vi "Write CurrentLeftMostItem.vi"(8 "error in (no error)":errorcluster, 10 "CurrentLeftMostItem":i32, 11 "BreadcrumbNavigation in":refnum<class "BreadcrumbNavigator.lvclass">) -> (0 "error out":errorcluster, 3 "BreadcrumbNavigation out":refnum<class "BreadcrumbNavigator.lvclass">)   [LabVIEW 2015, in "BreadcrumbNavigator.lvclass"]
uses:
  BreadcrumbNavigator.lvclass
  BreadcrumbNavigator.lvclass/BreadcrumbNavigator.ctl
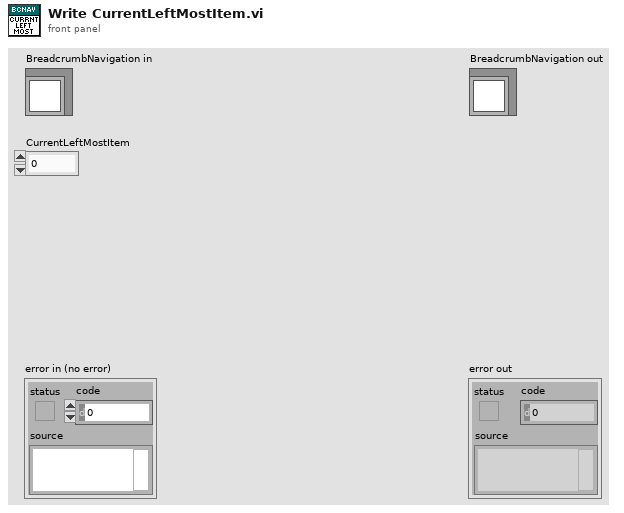
[diagram p1: front panel]
types:
  T1 = typedef "BreadcrumbNavigation.lvclass/State Data.ctl" = cluster{"Strings[]":string[], "CurrentLeftMostItem":i32, "Delimeter":string}
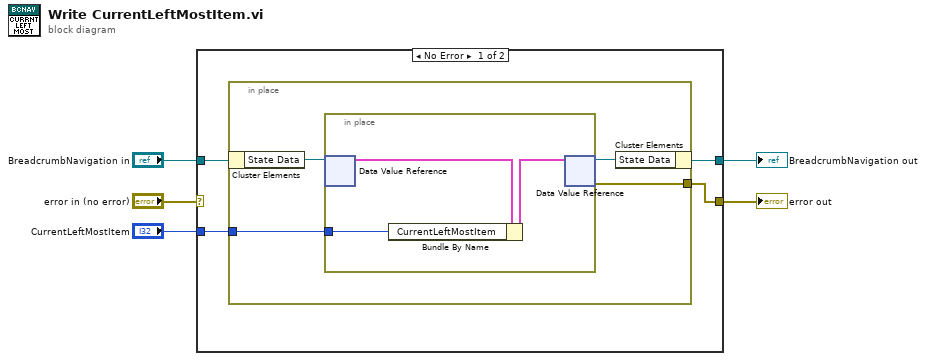
[diagram p0: block diagram]
diagram:
  n1 = case shown="No Error" "error in (no error)" {
    selector: "error in (no error)" -> [_ w18]
    tunnel: [w7 w18] -> w4
    tunnel: [w6 w17] -> w2
    tunnel: "BreadcrumbNavigation in" -> [w9 w17]
    tunnel: "CurrentLeftMostItem" -> [w8 _]
    frame No Error {
      n2 = in-place {
        in-place-border: w8 -> [w12]
        in-place-border: [w11] -> w7
        n3 = in-place-cluster #1(w9) -> ("State Data"=w13:refnum<data-value>)
        n4 = in-place {
          in-place-border: w12 -> [w14]
          n5 = in-place-dvr #2(w13) -> (w16:T1)  [unwired: 1 out]
          n6 = Bundle By Name(cluster=w16, "CurrentLeftMostItem"=w14) -> (w15:T1)
          n7 = in-place-dvr #2(w15) -> (w10:refnum<data-value>, w11:errorcluster)
        }
        n8 = in-place-cluster #1("State Data"=w10) -> (w6:refnum<class "BreadcrumbNavigator.lvclass">)
      }
    }
    frame Error {
    }
  }
  "error out" <- w4
  "BreadcrumbNavigation out" <- w2
